vi "FittingRange_Clipping.vi"(0 "Array in (X)":i32[](array[numeric]), 1 "L0 DAC":i32, 2 "IPR":i32, 3 "upper limit":dbl=0.8, 5 "Array in (Y)":i32[](array[numeric]), 7 "Array Pointer in":i32, 9 "Cycles Burst":i32=10000, 11 "error in":errorcluster, 12 "State machine":i32, 13 "lower limit":dbl=0.2) -> (4 "Array out (X)":i32[](array[numeric]), 6 "Array out (Y)":i32[](array[numeric]), 8 "Array Pointer out":i32, 10 "N_Array Elements":i32, 14 "State machine":i32, 15 "error out":errorcluster)   [LabVIEW 2009]
doc: "This VI collects the L0 DAC values that gives an IPR between the 80%-20% of the generated pulses."
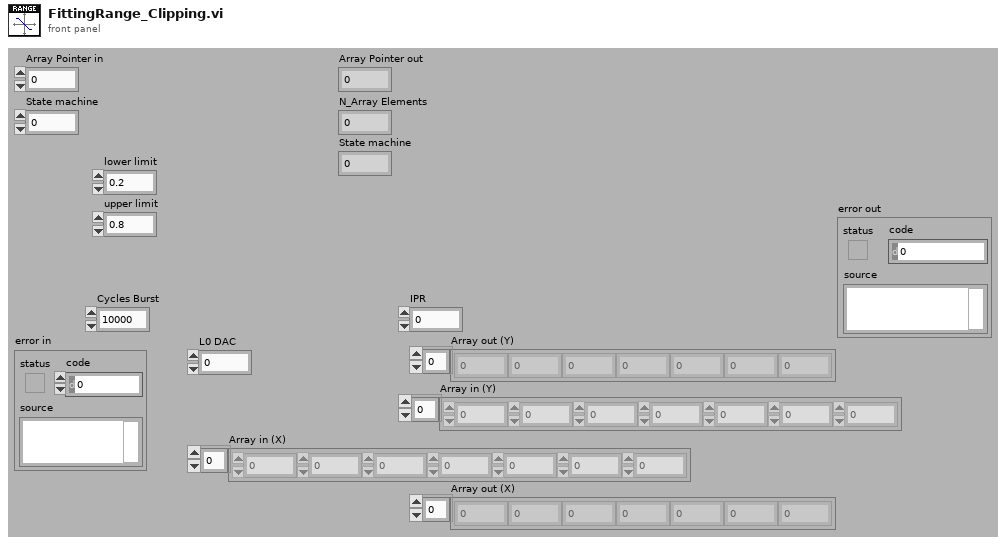
[diagram p1: front panel]
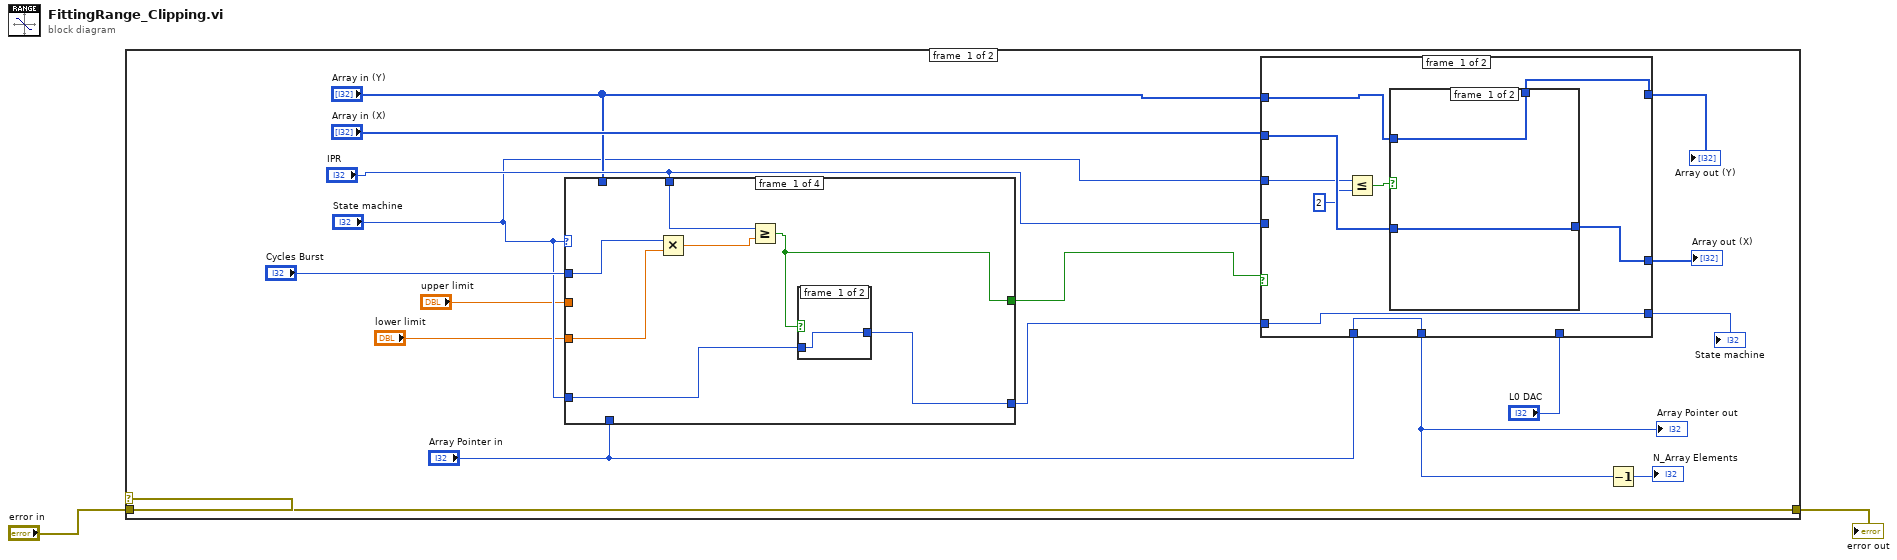
[diagram p0: block diagram]
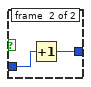
[diagram p2: hidden frame]
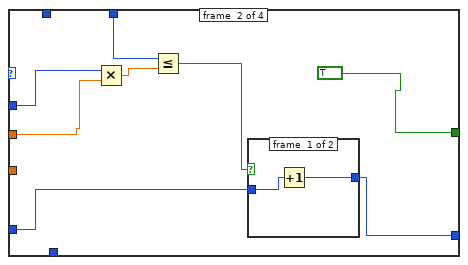
[diagram p3: hidden frame]
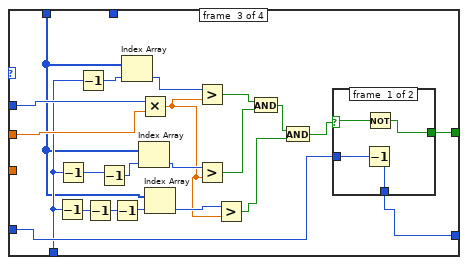
[diagram p5: hidden frame]
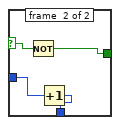
[diagram p6: hidden frame]
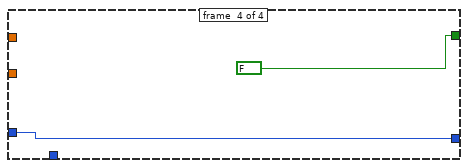
[diagram p7: hidden frame]
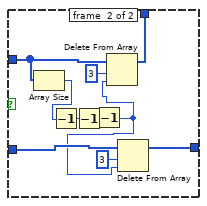
[diagram p8: hidden frame]
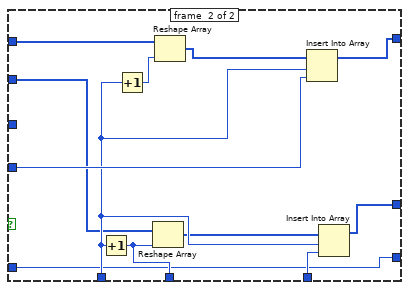
[diagram p9: hidden frame]
diagram:
  n1 = case shown="No Error" "error in" {
    tunnel: "error in" -> [w15 w106]
    tunnel: [w15 w106] -> w1
    frame #0 {
      n2 = case shown="2" "State machine" {
        tunnel: "Cycles Burst" -> [w25 w35 w62 _]
        tunnel: "IPR" -> [w24 w36 _ _]
        tunnel: "State machine" -> [w23 w33 w56 w72]
        tunnel: [w22 w34 w57 w72] -> w8
        tunnel: "Array in (Y)" -> [_ _ w45 _]
        tunnel: "Array Pointer in" -> [_ _ w46 _]
        tunnel: [w21 TRUE w52 FALSE ("record")] -> w5
        tunnel: "lower limit" -> [w20 _ _ _]
        tunnel: "upper limit" -> [_ w30 w51 _]
        frame #0 {
          n3 = Multiply(x=w25, y=w20) -> (x*y=w26:dbl)
          n4 = Greater Or Equal?(x=w24, y=w26) -> (x >= y?=w21:bool)
          n5 = case shown="True" w21 {
            tunnel: w23 -> [w27 w29]
            tunnel: [w27 w28] -> w22
            frame #0 {
            }
            frame #1 {
              n6 = Increment(x=w29) -> (x+1=w28:i32)
            }
          }
        }
        frame #1 {
          n7 = Multiply(x=w35, y=w30) -> (x*y=w37:dbl)
          n8 = Less Or Equal?(x=w36, y=w37) -> (x <= y?=w32:bool)
          n9 = case shown="False" w32 {
            tunnel: [w39 w40] -> w34
            tunnel: w33 -> [w38 w40]
            frame #0 {
              n10 = Increment(x=w38) -> (x+1=w39:i32)
            }
            frame #1 {
            }
          }
        }
        frame #2 {
          n11 = Decrement(x=w46) -> (x-1=w47:i32)
          n12 = Decrement(x=w46) -> (x-1=w55:i32)
          n13 = Decrement(x=w46) -> (x-1=w53:i32)
          n14 = Decrement(x=w47) -> (x-1=w48:i32)
          n15 = Decrement(x=w55) -> (x-1=w54:i32)
          n16 = Decrement(x=w48) -> (x-1=w49:i32)
          n17 = Index Array(array=w45, index=w53) -> (element=w61:i32)
          n18 = Index Array(array=w45, index=w54) -> (element=w59:i32)
          n19 = Multiply(x=w62, y=w51) -> (x*y=w44:dbl)
          n20 = Index Array(array=w45, index=w49) -> (element=w50:i32)
          n21 = Greater?(x=w61, y=w44) -> (0:w60:bool)
          n22 = Greater?(x=w59, y=w44) -> (0:w58:bool)
          n23 = Greater?(x=w50, y=w44) -> (0:w43:bool)
          n24 = And(x=w60, y=w58) -> (x .and. y?=w42:bool)
          n25 = And(x=w42, y=w43) -> (x .and. y?=w41:bool)
          n26 = case shown="True" w41 {
            selector: w41 -> [w63 w67]
            tunnel: [w66 w70] -> w57
            tunnel: w56 -> [w65 w69]
            tunnel: [w64 w68] -> w52
            frame #0 {
              n27 = Decrement(x=w65) -> (x-1=w66:i32)
              n28 = Not(x=w63) -> (.not. x?=w64:bool)
            }
            frame #1 {
              n29 = Not(x=w67) -> (.not. x?=w68:bool)
              n30 = Increment(x=w69) -> (x+1=w70:i32)
            }
          }
        }
        frame #3 {
        }
      }
      n31 = case shown="False" w5 {
        tunnel: "IPR" -> [_ w105]
        tunnel: [w78 w99] -> w19
        tunnel: "Array in (Y)" -> [w79 w101]
        tunnel: "L0 DAC" -> [_ w104]
        tunnel: "Array in (X)" -> [w76 w95]
        tunnel: [w77 w96] -> w16
        tunnel: "Array Pointer in" -> [w81 w98]
        tunnel: [w81 w102] -> w13
        tunnel: w8 -> [w80 w94]
        tunnel: [w80 w94] -> w7
        tunnel: "State machine" -> [w74 _]
        frame #0 {
          n32 = Less Or Equal?(x=w74, y=2) -> (x <= y?=w75:bool)
          n33 = case shown="True" w75 {
            tunnel: w79 -> [w83 w93]
            tunnel: [w83 w88] -> w78
            tunnel: [w82 w86] -> w77
            tunnel: w76 -> [w82 w85]
            frame #0 {
            }
            frame #1 {
              n34 = Array Size(array=w93) -> (size(s)=w92:i32)
              n35 = Decrement(x=w92) -> (x-1=w91:i32)
              n36 = Decrement(x=w91) -> (x-1=w90:i32)
              n37 = Decrement(x=w90) -> (x-1=w84:i32)
              n38 = Delete From Array(array=w93, length=3, index=w84) -> (array with subset deleted=w88:i32[])  [unwired: 1 out]
              n39 = Delete From Array(array=w85, length=3, index=w84) -> (array with subset deleted=w86:i32[])  [unwired: 1 out]
            }
          }
        }
        frame #1 {
          n40 = Increment(x=w98) -> (x+1=w102:i32)
          n41 = Increment(x=w98) -> (x+1=w103:i32)
          n42 = Reshape Array(w95, w102) -> (w97:i32[])
          n43 = Reshape Array(w101, w103) -> (w100:i32[])
          n44 = Insert Into Array(array=w100, index=w98, new element=w105) -> (w99:i32[])
          n45 = Insert Into Array(array=w97, index=w98, new element=w104) -> (w96:i32[])
        }
      }
      "Array out (Y)" <- w19
      "Array out (X)" <- w16
      "Array Pointer out" <- w13
      "State machine" <- w7
      n46 = Decrement(x=w13) -> (x-1=→"N_Array Elements":i32)
    }
    frame #1 {
    }
  }
  "error out" <- w1
